vi "obtain_instrument_name.vi"(3 "input_machine_reference.lvclass":refnum<class "machine.lvclass">) -> (1 "output_machine_reference.lvclass":refnum<class "machine.lvclass">)   [LabVIEW 2014, in "machine.lvclass"]
uses:
  machine.lvclass
  machine.lvclass/machine.ctl
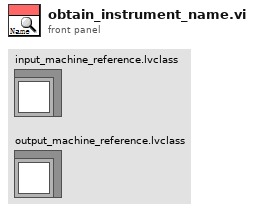
[diagram p1: front panel]
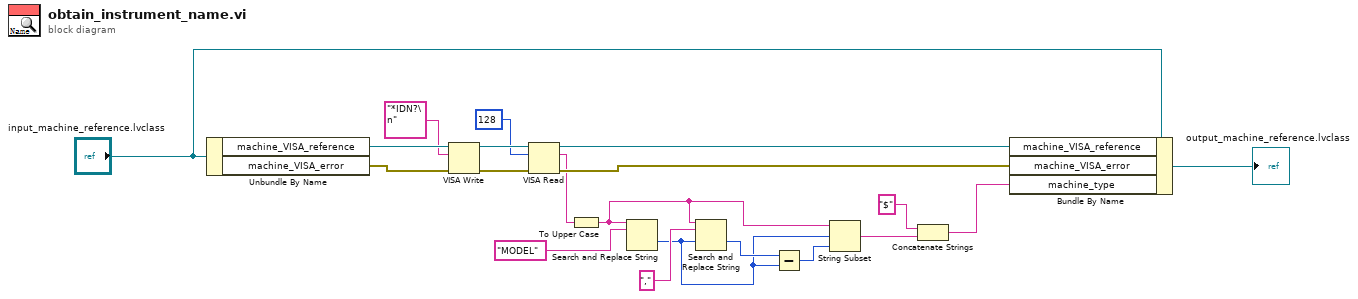
[diagram p0: block diagram]
diagram:
  n1 = Unbundle By Name("input_machine_reference.lvclass") -> ("machine_VISA_reference"=w18:refnum<visa-resource-name>, "machine_VISA_error"=w17:errorcluster)
  n2 = VISA Write(VISA resource name=w18, write buffer="*IDN?\n", error in (no error)=w17) -> (VISA resource name out=w15:refnum<visa-resource-name>, error out=w14:errorcluster)  [unwired: 1 out]
  n3 = VISA Read(VISA resource name=w15, byte count=u32 128, error in (no error)=w14) -> (VISA resource name out=w12:refnum<visa-resource-name>, read buffer=w10:string, error out=w11:errorcluster)  [unwired: 1 out]
  n4 = To Upper Case(1:w10) -> (0:w7:string)
  n5 = Search and Replace String(input string=w7, search string="MODEL") -> (offset past replacement=w5:i32)  [unwired: 6 in, 3 out]
  n6 = Search and Replace String(input string=w7, search string=",", offset=w5) -> (offset past replacement=w6:i32)  [unwired: 5 in, 3 out]
  n7 = Subtract(x=w6, y=w5) -> (x-y=w4:i32)
  n8 = String Subset(string=w7, offset (0)=w5, length (rest)=w4) -> (substring=w3:string)
  n9 = Concatenate Strings("$" ("string"), w3) -> (w1:string)
  n10 = Bundle By Name(cluster="input_machine_reference.lvclass", "machine_VISA_reference"=w12, "machine_VISA_error"=w11, "machine_type"=w1) -> (→"output_machine_reference.lvclass":refnum<class "machine.lvclass">)
